vi "Emballage_bdd_recherche_toutes_les Correspondance.vi"(9 "tableau des codes barres":string[](array[string]), 10 "1er index":i32, 11 "Sous_chaine":string) -> (3 "Tableau_Indice":i32[](array[numeric]))   [LabVIEW 2020]
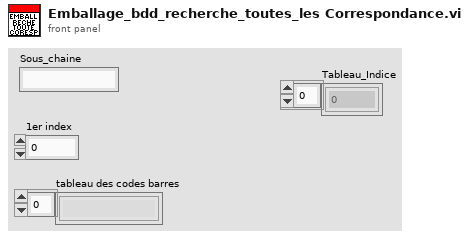
[diagram p1: front panel]
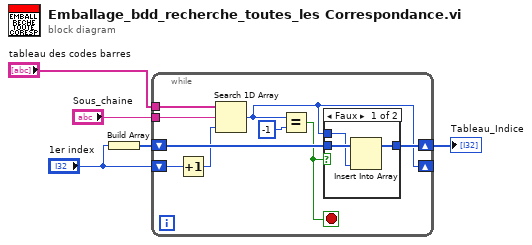
[diagram p0: block diagram]
diagram:
  n1 = Build Array("1er index") -> (w2:i32[])
  n2 = while {
    shift-right: [w13] -> w5
    shift-left: w2 -> [w14]
    tunnel: "tableau des codes barres" -> [w12]
    shift-right: [w9] -> _
    shift-left: "1er index" -> [w11]
    tunnel: "Sous_chaine" -> [w7]
    stop <- w8 stop-if-true
    n3 = Increment(x=w11) -> (x+1=w6:i32)
    n4 = Search 1D Array(1D array=w12, element=w7, start index (0)=w6) -> (index of element=w9:i32)
    n5 = Equal?(x=w9, y=-1) -> (x = y?=w8:bool)
    n6 = case shown="Faux" w8 {
      tunnel: w14 -> [w17 w18]
      tunnel: [w16 w18] -> w13
      tunnel: w9 -> [w15 _]
      frame False {
        n7 = Insert Into Array(array=w17, new element=w15) -> (w16:i32[])  [unwired: 1 in]
      }
      frame True {
      }
    }
  }
  "Tableau_Indice" <- w5
